vi "Root Directory.vi"() -> (0 "Root Directory":string="/", 1 "Directory Tree":T1)   [LabVIEW 2020, in "AoC 2022.lvlib"]
uses:
  AoC 2022.lvlib
  Directory Tree.ctl
  Directory Contents.ctl
  File.ctl
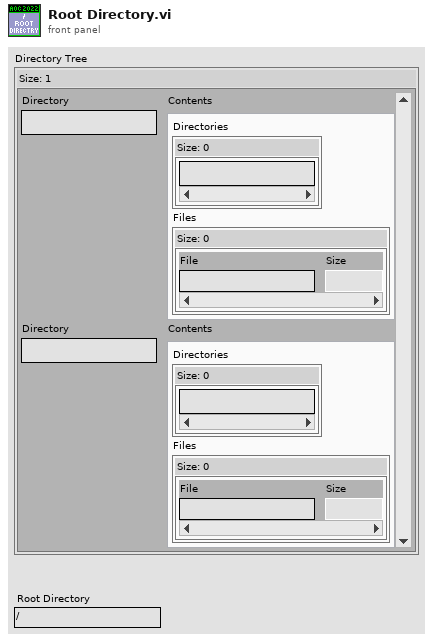
[diagram p1: front panel]
types:
  T1 = typedef "AoC 2022.lvlib/Directory Tree.ctl" = map{string, T2}
  T2 = typedef "AoC 2022.lvlib/Directory Contents.ctl" = cluster{"Directories":set{string}, "Files":T3}
  T3 = typedef "AoC 2022.lvlib/File.ctl" = map{string, u64}
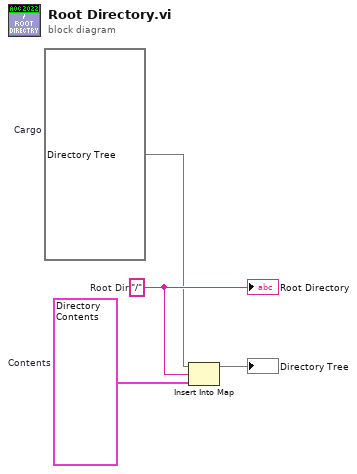
[diagram p0: block diagram]
diagram:
  w3 = "/"  # Root Dir
  w2 = T2 {"Directories"={}, "Files"={}}  # Contents
  w1 = T1 {}  # Cargo
  n1 = Insert Into Map(map in=w1, key=w3, value=w2) -> (map out=→"Directory Tree":T1)  [unwired: 2 out]
  "Root Directory" <- w3
